vi "InitializeQueue.vi"(8 "error in (no error)":errorcluster, 9 "taskId":i32(ring)=1 items=["TLibrary", "T01", "T02", "T03", "T04", "T05", "T06", "T07", "T08", "T09", "T10", "T11", "T12", "T13", "T14", "T15", "T16", "T17", "T18", "T19", "T20", "T21", "T22", "T23", "T24", "T25", "T26", "T27", "T28", "T29", "T30", "T31"], 11 "controller in":refnum<k24>) -> (0 "error out":errorcluster, 3 "controller out":refnum<k24>)   [LabVIEW 2021]
uses:
  C:/Program Files (x86)/Aerotech/A3200/LabVIEW/2010/Bin/Aerotech.A3200.dll
  Bin/Aerotech.A3200.dll
  C:/Program Files (x86)/Aerotech/A3200/LabVIEW/2010/Bin/Aerotech.A3200.LabVIEW.dll
  Bin/Aerotech.A3200.LabVIEW.dll
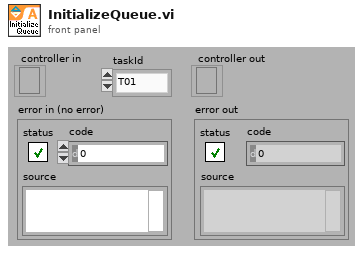
[diagram p1: front panel]
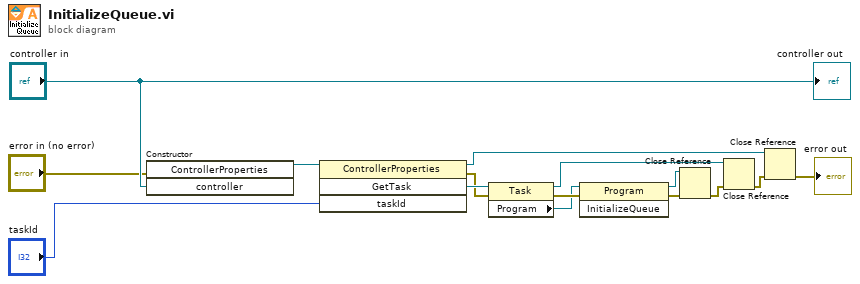
[diagram p0: block diagram]
diagram:
  n1 = constructor class="ControllerProperties"(error in="error in (no error)", "controller"="controller in") -> (reference out=w13:refnum<k24>)  [unwired: 2 in, 3 out]
  n2 = invoke class="ControllerProperties" method="GetTask"(reference=w13, "taskId"="taskId") -> (reference out=w2:refnum<k24>, error out=w10:errorcluster, "GetTask"=w11:refnum<k24>)  [unwired: 2 in, 1 out]
  n3 = property class="Task"(reference=w11, error in=w10) -> (reference out=w4:refnum<k24>, error out=w9:errorcluster, "Program"=w8:refnum<k24>)
  n4 = invoke class="Program" method="InitializeQueue"(reference=w8, error in=w9) -> (reference out=w6:refnum<k24>, error out=w7:errorcluster)  [unwired: 1 in, 1 out]
  n5 = Close Reference(reference=w6, error in (no error)=w7) -> (error out=w5:errorcluster)
  n6 = Close Reference(reference=w4, error in (no error)=w5) -> (error out=w3:errorcluster)
  n7 = Close Reference(reference=w2, error in (no error)=w3) -> (error out=→"error out":errorcluster)
  "controller out" <- "controller in"
